vi "Main.vi"(11 "Error In":errorcluster) -> (15 "Error Out":errorcluster)   [LabVIEW 2023]
uses:
  Controls/Queue Operation.ctl
  Controls/User Event Operations.ctl
  Classes/User Sender/Methods/Sender UI.vi
  Classes/User Receiver/Methods/Receiver UI.vi
  Classes/User Sender/User Sender.lvclass
  Classes/User Receiver/User Receiver.lvclass
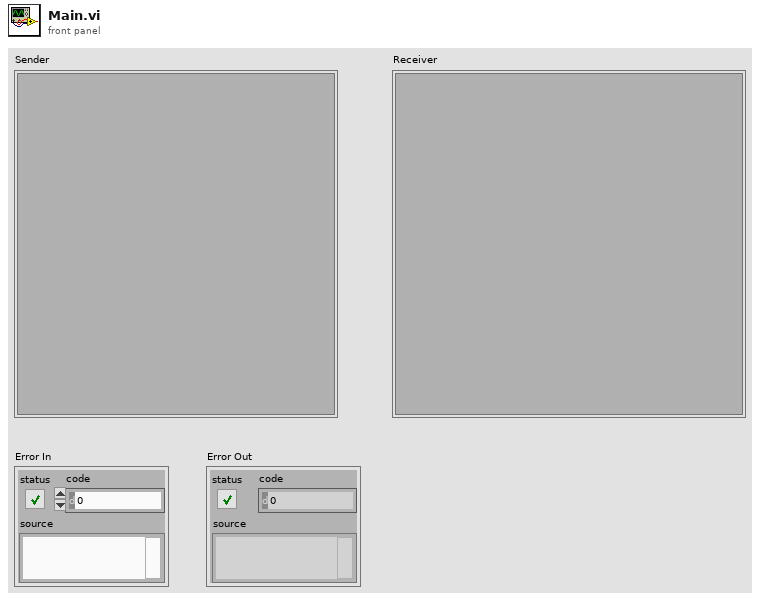
[diagram p1: front panel]
types:
  T1 = typedef "User Event Operations.ctl" = enum16{"Obtain", "Generate", "Destroy"}
  T2 = typedef "Queue Operation.ctl" = enum16{"Create & Enqueue N", "Enqueue N", "Dequeue", "Enstack N", "Flush", "Release"}
  T3 = typedef "Queue Element.ctl" = cluster{"State":string, "Data":variant}
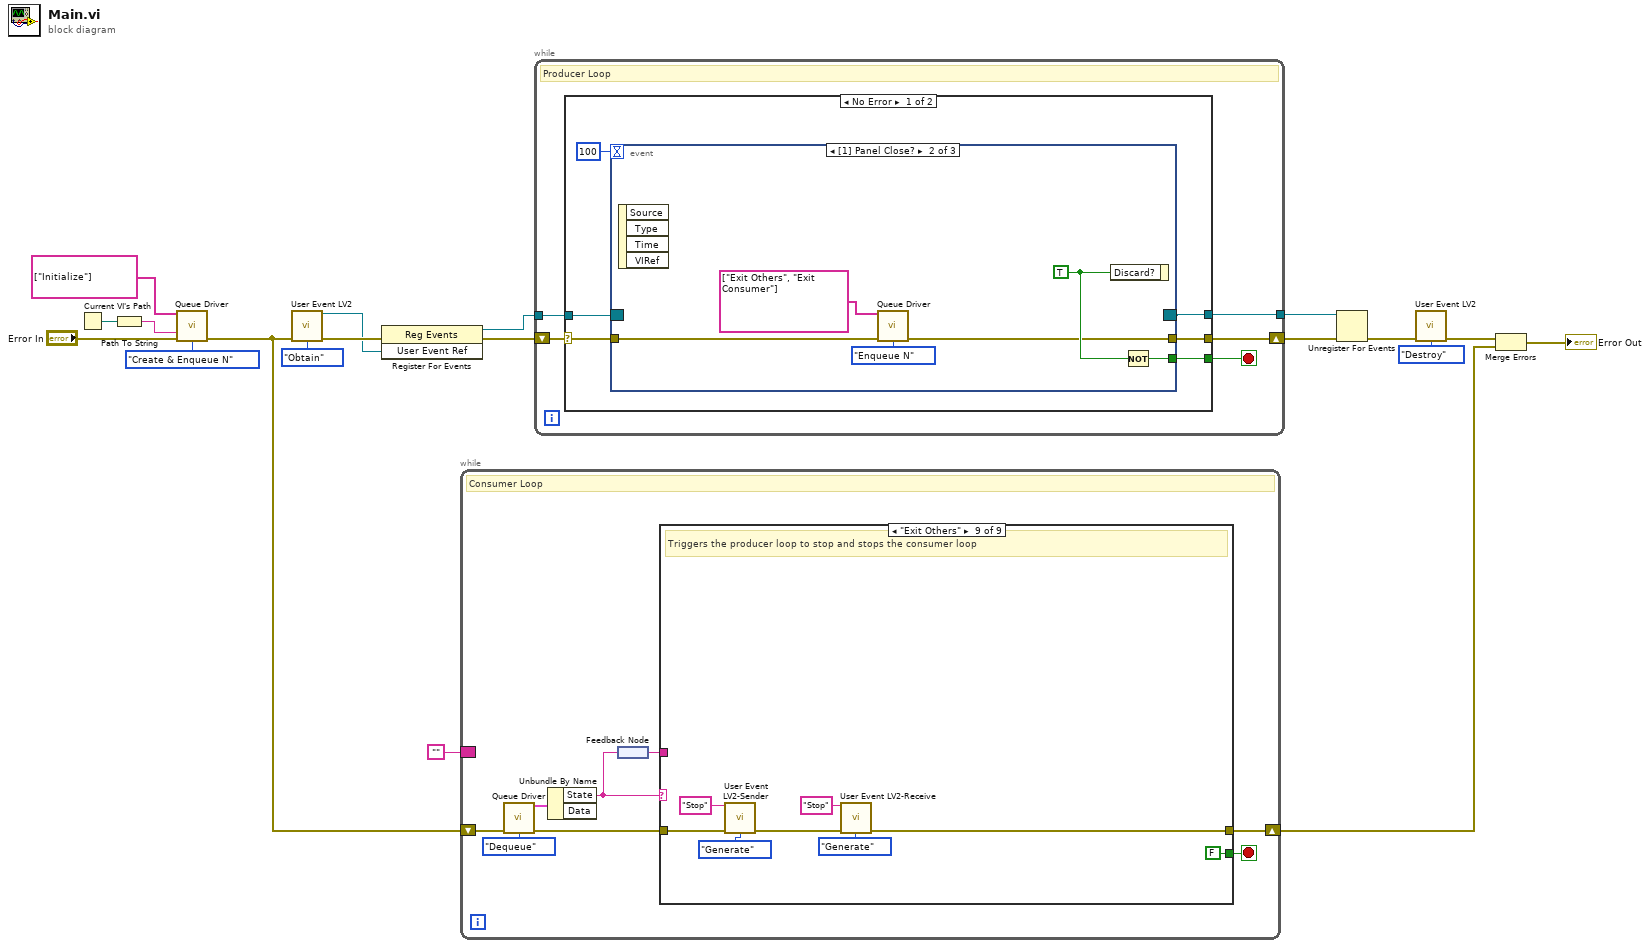
[diagram p0: block diagram]
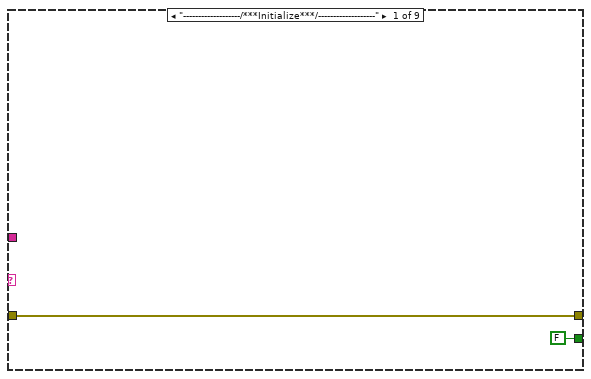
[diagram p2: hidden frame]
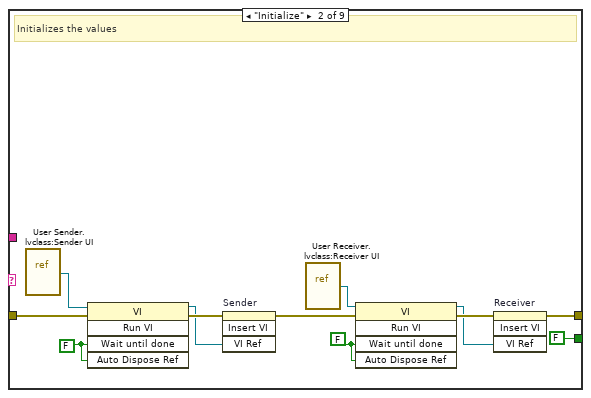
[diagram p3: hidden frame]
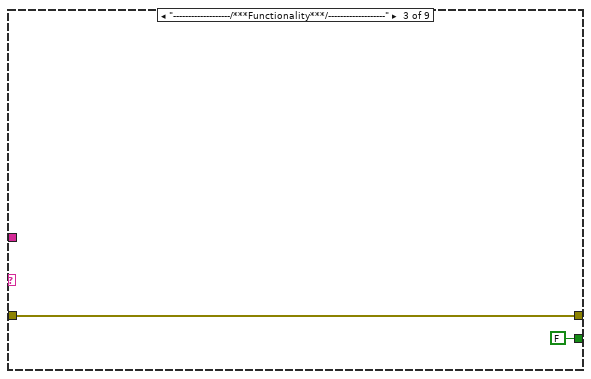
[diagram p4: hidden frame]
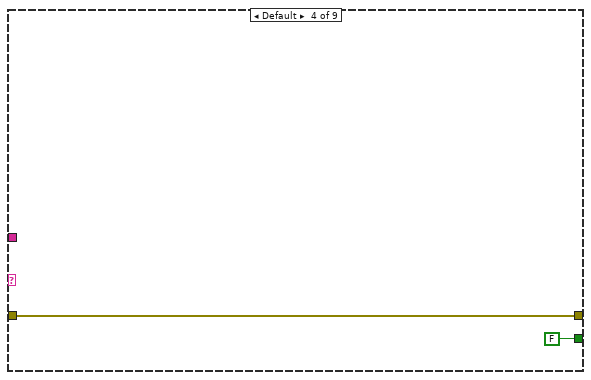
[diagram p5: hidden frame]
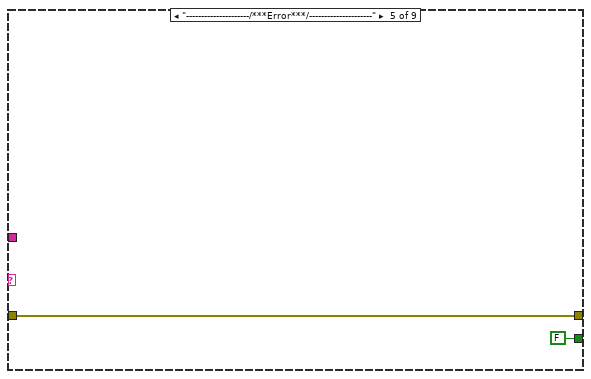
[diagram p6: hidden frame]
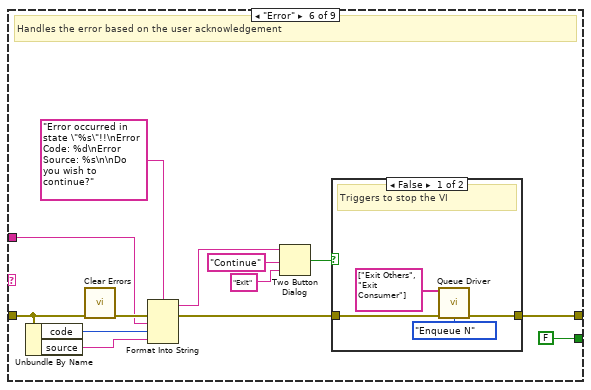
[diagram p7: hidden frame]
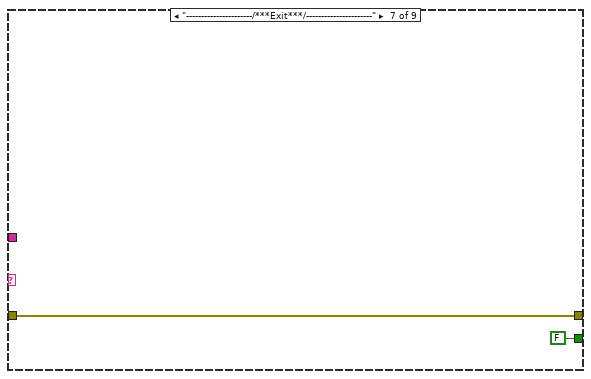
[diagram p9: hidden frame]
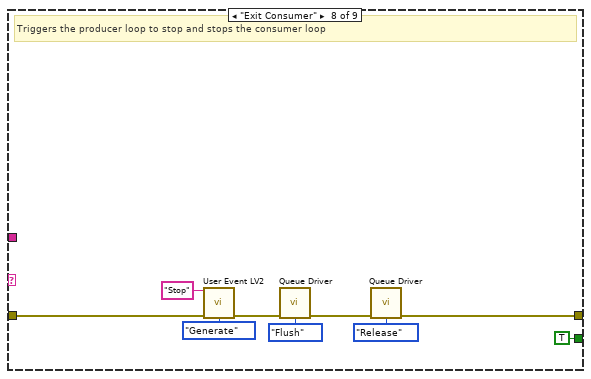
[diagram p10: hidden frame]
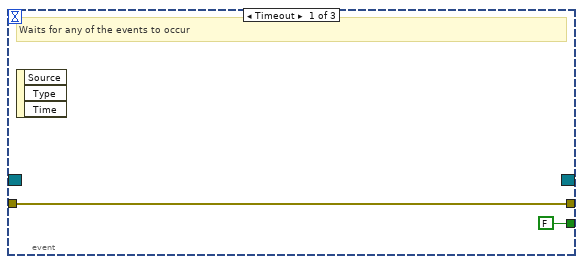
[diagram p11: hidden frame]
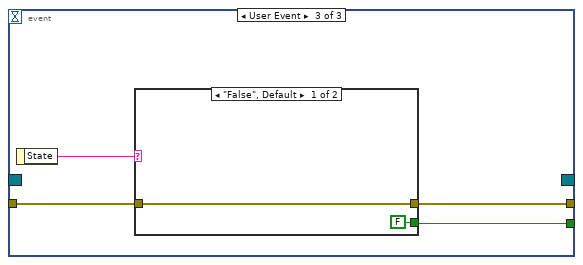
[diagram p12: hidden frame]
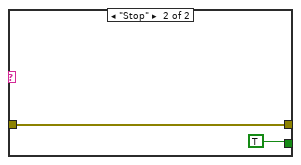
[diagram p13: hidden frame]
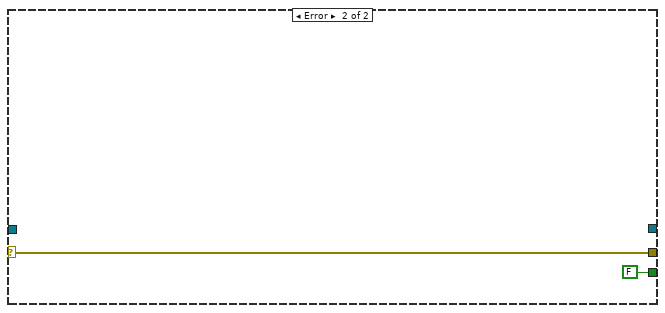
[diagram p14: hidden frame]
diagram:
  n1 = Current VI's Path() -> (path=w16:path)
  n2 = Path To String(path=w16) -> (string=w15:string)
  n3 = call "Queue Driver.vi"("States[]"=string[] ["Initialize"], "Queue Name"=w15, "Error In"="Error In", "Queue Operation"=Queue_Operation."Create & Enqueue N") -> ("Error Out"=w9:errorcluster)  [unwired: 10 in, 1 out]
  n4 = call "User Event LV2.vi"("Error In"=w9, "Operation"=User_Event_Operations."Obtain") -> ("User Event Ref"=w7:refnum<user-event>, "Error Out"=w11:errorcluster)  [unwired: 12 in]
  n5 = register-events(error in=w11, w7) -> (reference out=w6:refnum<event-registration>, error out=w8:errorcluster)  [unwired: 1 in]
  n6 = while {
    shift-right: [w26] -> w12
    shift-left: w9 -> [w27]
    border: "" -> [_]
    stop <- w22 stop-if-true
    # "Consumer Loop"
    n7 = call "Queue Driver.vi"("Error In"=w27, "Queue Operation"=Queue_Operation."Dequeue") -> ("Dequeue Element"=w23:T3, "Error Out"=w25:errorcluster)  [unwired: 12 in]
    n8 = Unbundle By Name(w23) -> ("State"=w21:string)  [unwired: 1 out]
    n9 = feedback-in #1(w21) -> ()
    n10 = feedback #1() -> (w20:string)
    n11 = case shown="\"Exit Others\"" w21 {
      tunnel: w25 -> [w29 w41 w43 w45 w47 w52 w67 w76 w84]
      tunnel: [w29 w33 w43 w45 w47 w49 w67 w72 w79] -> w26
      tunnel: [FALSE FALSE FALSE FALSE FALSE FALSE FALSE TRUE FALSE] -> w22
      tunnel: w20 -> [_ _ _ _ _ w50 _ _ _]
      frame "-------------------/***Initialize***/-------------------" {
      }
      frame "Initialize" {
        w36 = FALSE ("Wait Until Done")
        w38 = FALSE ("Wait Until Done")
        # "Initializes the values"
        n12 = vi-ref "User Sender.lvclass:Sender UI.vi"() -> (w39:refnum<vi>)
        n13 = invoke class="VI" method="Run VI"(reference=w39, error in=w41, "Wait until done"=w38, "Auto Dispose Ref"=w38) -> (reference out=w30:refnum<vi>, error out=w32:errorcluster)  [unwired: 1 in, 3 out]
        n14 = invoke on="Sender" class="SubPnl" method="Insert VI"(error in=w32, "VI Ref"=w30) -> (error out=w31:errorcluster)  [unwired: 2 in, 3 out]
        n15 = vi-ref "User Receiver.lvclass:Receiver UI.vi"() -> (w37:refnum<vi>)
        n16 = invoke class="VI" method="Run VI"(reference=w37, error in=w31, "Wait until done"=w36, "Auto Dispose Ref"=w36) -> (reference out=w34:refnum<vi>, error out=w35:errorcluster)  [unwired: 1 in, 3 out]
        n17 = invoke on="Receiver" class="SubPnl" method="Insert VI"(error in=w35, "VI Ref"=w34) -> (error out=w33:errorcluster)  [unwired: 2 in, 3 out]
      }
      frame "-------------------/***Functionality***/-------------------" {
      }
      frame Default {
      }
      frame "---------------------/***Error***/---------------------" {
      }
      frame "Error" {
        # "Handles the error based on the user acknowledgement"
        n18 = Unbundle By Name(w52) -> ("code"=w54:i32, "source"=w53:string)
        n19 = call <vilib>:"Clear Errors.vi"("error in (no error)"=w52) -> ("error out"=w59:errorcluster)  [unwired: 5 in, 1 out]
        n20 = Format Into String(format string="Error occurred in state \"%s\"!!\nError Code: %d\nError Source: %s\n\nDo you wish to continue?", error in=w59, w50, w54, w53) -> (resulting string=w57:string, error out=w51:errorcluster)  [unwired: 1 in]
        n21 = Two Button Dialog(message=w57, 1:"Exit" ("F button name (\"Cancel\")"), 2:"Continue" ("T button name (\"OK\")")) -> (T button?=w48:bool)
        n22 = case shown="False" w48 {
          tunnel: w51 -> [w64 w65]
          tunnel: [w63 w65] -> w49
          frame False {
            # "Triggers to stop the VI"
            n23 = call "Queue Driver.vi"("States[]"=string[] ["Exit Others", "Exit Consumer"], "Error In"=w64, "Queue Operation"=Queue_Operation."Enqueue N") -> ("Error Out"=w63:errorcluster)  [unwired: 11 in, 1 out]
          }
          frame True {
          }
        }
      }
      frame "----------------------/***Exit***/----------------------" {
      }
      frame "Exit Consumer" {
        # "Triggers the producer loop to stop and stops the consumer loop"
        n24 = call "User Event LV2.vi"("Event Name"="Stop", "Error In"=w76, "Operation"=User_Event_Operations."Generate") -> ("Error Out"=w70:errorcluster)  [unwired: 11 in, 1 out]
        n25 = call "Queue Driver.vi"("Error In"=w70, "Queue Operation"=Queue_Operation."Flush") -> ("Error Out"=w74:errorcluster)  [unwired: 12 in, 1 out]
        n26 = call "Queue Driver.vi"("Error In"=w74, "Queue Operation"=Queue_Operation."Release") -> ("Error Out"=w72:errorcluster)  [unwired: 12 in, 1 out]
      }
      frame "Exit Others" {
        # "Triggers the producer loop to stop and stops the consumer loop"
        n27 = call "User Event LV2-Sender.vi"("Event Name"="Stop", "Error In"=w84, "Operation"=User_Event_Operations."Generate") -> ("Error Out"=w82:errorcluster)  [unwired: 11 in, 1 out]
        n28 = call "User Event LV2-Receive.vi"("Event Name"="Stop", "Error In"=w82, "Operation"=User_Event_Operations."Generate") -> ("Error Out"=w79:errorcluster)  [unwired: 11 in, 1 out]
      }
    }
  }
  n29 = while {
    shift-right: [w87] -> w18
    shift-left: w8 -> [w88]
    tunnel: w6 -> [w86]
    tunnel: [w85] -> w4
    stop <- w89 stop-if-true
    # "Producer Loop"
    n30 = case shown="No Error" w88 {
      selector: w88 -> [w94 w113]
      tunnel: [w95 FALSE] -> w89
      tunnel: [w93 w113] -> w87
      tunnel: w86 -> [w91 _]
      tunnel: [w90 _] -> w85
      frame No Error {
        n31 = event shown="[1] Panel Close?" {
          selector: w91 -> [_ _ _]
          dyn-events: [_ _ _] -> w90
          timeout: 100 -> [_ _ _]
          tunnel: [FALSE w102 w104] -> w95
          tunnel: w94 -> [w96 w101 w107]
          tunnel: [w96 w100 w106] -> w93
          event Timeout {
            # "Waits for any of the events to occur"
            n32 = event-data() -> ()  [unwired: 1 in, 3 out]
          }
          event Panel Close? {
            w103 = TRUE ("Discard?")
            n33 = event-data() -> ()  [unwired: 1 in, 4 out]
            n34 = call "Queue Driver.vi"("States[]"=string[] ["Exit Others", "Exit Consumer"], "Error In"=w101, "Queue Operation"=Queue_Operation."Enqueue N") -> ("Error Out"=w100:errorcluster)  [unwired: 11 in, 1 out]
            n35 = event-data("Discard?"=w103) -> ()  [unwired: 1 in, 1 out]
            n36 = Not(x=w103) -> (.not. x?=w102:bool)
          }
          event User Event {
            n37 = event-data() -> ("State"=w105:string)  [unwired: 1 in]
            n38 = case shown="\"False\", Default" w105 {
              tunnel: w107 -> [w109 w111]
              tunnel: [w109 w111] -> w106
              tunnel: [FALSE TRUE] -> w104
              frame "False", Default {
              }
              frame "Stop" {
              }
            }
          }
        }
      }
      frame Error {
      }
    }
  }
  n39 = Unregister For Events(event registration refnum=w4, error in=w18) -> (error out=w5:errorcluster)
  n40 = call "User Event LV2.vi"("Error In"=w5, "Operation"=User_Event_Operations."Destroy") -> ("Error Out"=w3:errorcluster)  [unwired: 12 in, 1 out]
  n41 = Merge Errors(w3, w12) -> (→"Error Out":errorcluster)
